vi "DelayPiezo.vi"(0 "old timer value":u32, 2 "milliseconds to wait":u32, 3 "error in (no error)":errorcluster) -> (6 "new time":u32, 7 "elapsed time":u32, 9 "error out":errorcluster)   [LabVIEW 2020]
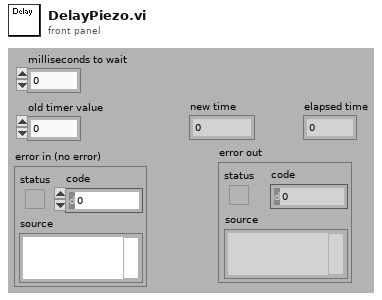
[diagram p1: front panel]
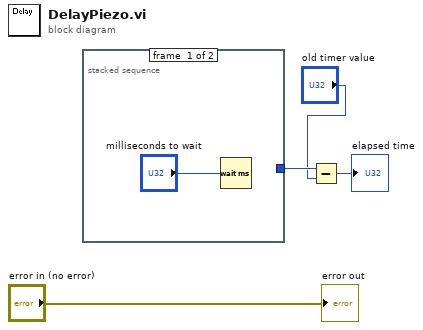
[diagram p0: block diagram]
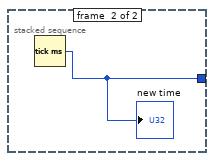
[diagram p2: hidden frame]
diagram:
  n1 = stacked-sequence {
    tunnel: [_ w6] -> w3
    frame #0 {
      n2 = Wait (ms)(milliseconds to wait="milliseconds to wait") -> ()  [unwired: 1 out]
    }
    frame #1 {
      n3 = Tick Count (ms)() -> (millisecond timer value=w6:u32)
      "new time" <- w6
    }
  }
  n4 = Subtract(x=w3, y="old timer value") -> (x-y=→"elapsed time":u32)
  "error out" <- "error in (no error)"
